vi "ReceiveMessage.vi"(8 "error in (no error)":errorcluster, 10 "BT Queue":refnum<queue>, 11 ".NET Refnum in":refnum<k24>) -> (0 "error out":errorcluster, 2 "String":string, 3 ".NET Refnum out":refnum<k24>)   [LabVIEW 2013, in "main.lvlib"]
uses:
  main.lvlib
  C:/Users/Simon/SkyDrive/LabView/2013/DM2020/bin/medimatic_bt_receiver.dll
  bin/medimatic_bt_receiver.dll
  Controls/Enum User Events.ctl
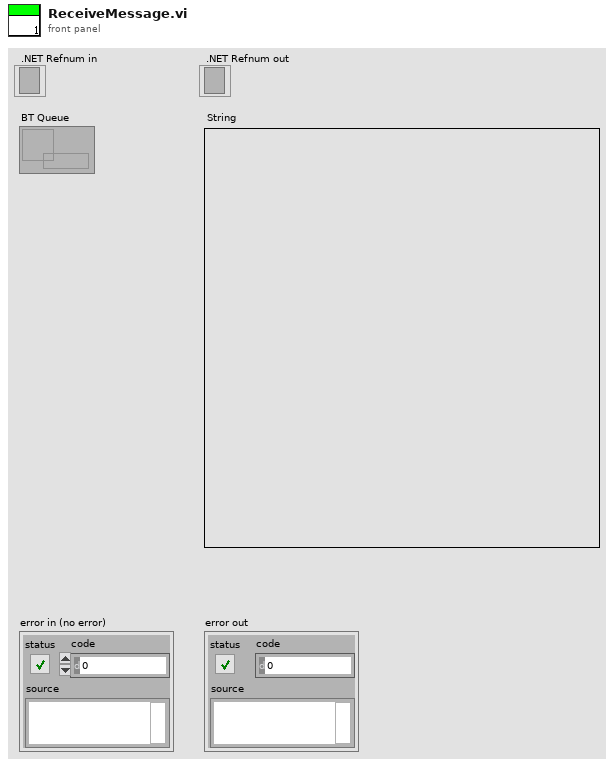
[diagram p1: front panel]
types:
  T1 = typedef "main.lvlib/Enum User Events.ctl" = enum16{"User Event", "Init"}
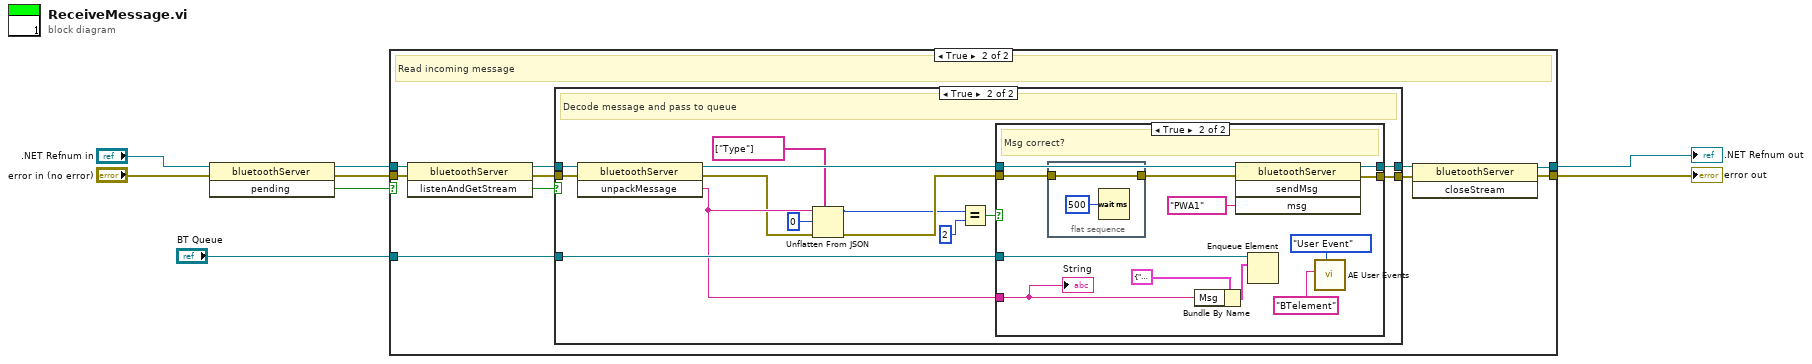
[diagram p0: block diagram]
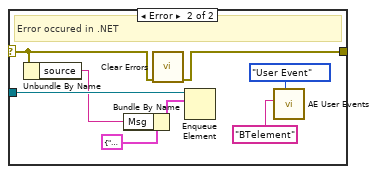
[diagram p5: hidden frame]
diagram:
  n1 = invoke class="bluetoothServer" method="pending"(reference=".NET Refnum in", error in="error in (no error)") -> (reference out=w7:refnum<k24>, error out=w6:errorcluster, "pending"=w8:bool)  [unwired: 1 in]
  n2 = case shown="True" w8 {
    tunnel: [w9 w14] -> w3
    tunnel: [w10 w13] -> w2
    tunnel: w6 -> [w10 w17]
    tunnel: w7 -> [w9 w16]
    tunnel: "BT Queue" -> [_ w11]
    frame False {
    }
    frame True {
      # "Read incoming message"
      n3 = invoke class="bluetoothServer" method="listenAndGetStream"(reference=w16, error in=w17) -> (reference out=w19:refnum<k24>, error out=w18:errorcluster, "listenAndGetStream"=w20:bool)  [unwired: 1 in]
      n4 = case shown="True" w20 {
        tunnel: w19 -> [w22 w36]
        tunnel: w18 -> [w21 w35]
        tunnel: w11 -> [_ w29]
        tunnel: [w22 w33] -> w15
        tunnel: [w21 w32] -> w12
        frame False {
        }
        frame True {
          # "Decode message and pass to queue"
          n5 = invoke class="bluetoothServer" method="unpackMessage"(reference=w36, error in=w35) -> (reference out=w34:refnum<k24>, error out=w27:errorcluster, "unpackMessage"=w28:string)  [unwired: 1 in]
          n6 = Unflatten From JSON(path=string[] ["Type"], JSON string=w28, type and defaults=0, error in (no error)=w27) -> (value=w23:i32, error out=w26:errorcluster)  [unwired: 3 in]
          n7 = Equal?(x=w23, y=2) -> (x = y?=w30:bool)
          n8 = case shown="True" w30 {
            tunnel: w34 -> [w40 w61]
            tunnel: w26 -> [w39 w52]
            tunnel: [w40 w59] -> w33
            tunnel: [w38 w58] -> w32
            tunnel: w29 -> [w37 w55]
            tunnel: w28 -> [_ w50]
            frame False {
              # "Check for error"
              n9 = case shown="No Error" w39 {
                selector: w39 -> [w41 w43]
                tunnel: [w41 w42] -> w38
                tunnel: w37 -> [_ w49]
                frame No Error {
                }
                frame Error {
                  # "Error occured in .NET"
                  n10 = Unbundle By Name(w43) -> ("source"=w45:string)
                  n11 = Bundle By Name(cluster=cluster{"Cmd":string, "Msg":string} {"Cmd"="Error", "Msg"=""}, "Msg"=w45) -> (w44:cluster{"Cmd":string, "Msg":string})
                  n12 = call <vilib>:"Clear Errors.vi"("error in (no error)"=w43) -> ("error out"=w42:errorcluster)  [unwired: 6 in]
                  n13 = Enqueue Element(queue=w49, element=w44) -> ()  [unwired: 2 in, 3 out]
                  n14 = call "AE User Events.vi"("Action"=Enum_User_Events."User Event", "User Event"="BTelement") -> ()  [unwired: 8 in, 2 out]
                }
              }
            }
            frame True {
              # "Msg correct?"
              n15 = flat-sequence {
                tunnel: w52 -> [w62]
                tunnel: [w62] -> w51
                frame #0 {
                  n16 = Wait (ms)(milliseconds to wait=u32 500) -> ()  [unwired: 1 out]
                }
              }
              n17 = Bundle By Name(cluster=cluster{"Cmd":string, "Msg":string} {"Cmd"="BTelement", "Msg"=""}, "Msg"=w50) -> (w57:cluster{"Cmd":string, "Msg":string})
              n18 = invoke class="bluetoothServer" method="sendMsg"(reference=w61, error in=w51, "msg"="PWA1") -> (reference out=w59:refnum<k24>, error out=w58:errorcluster)  [unwired: 1 in, 2 out]
              n19 = Enqueue Element(queue=w55, element=w57) -> ()  [unwired: 2 in, 3 out]
              n20 = call "AE User Events.vi"("Action"=Enum_User_Events."User Event", "User Event"="BTelement") -> ()  [unwired: 8 in, 2 out]
              "String" <- w50
            }
          }
        }
      }
      n21 = invoke class="bluetoothServer" method="closeStream"(reference=w15, error in=w12) -> (reference out=w14:refnum<k24>, error out=w13:errorcluster)  [unwired: 1 in, 1 out]
    }
  }
  "error out" <- w2
  ".NET Refnum out" <- w3
